vi "gui_config.vi"(0 "PS Setting":T2, 1 "LIMIT":T1, 5 "error in (no error)":errorcluster, 6 "Torque":refnum<vi>, 12 "Speed":refnum<vi>) -> (11 "Water mode":bool, 13 "Offset out":dbl, 14 "PS Setting out":T2, 15 "Set_ECU_MODE":i32, 16 "mode out":bool, 17 "LIMIT  out":T1, 18 "power mode":bool, 19 "error out":errorcluster)   [LabVIEW 2019]
uses:
  ps_setting.ctl
  LIMIT DATA.ctl
panel:
  in  "Offset":dbl
  in  "chiller":bool
  in  "ps":bool
  in  "mode":bool
  in  "Exit":bool
  in  "最高转速 [rpm]":i32
  in  "最大扭矩 [Nm]":dbl
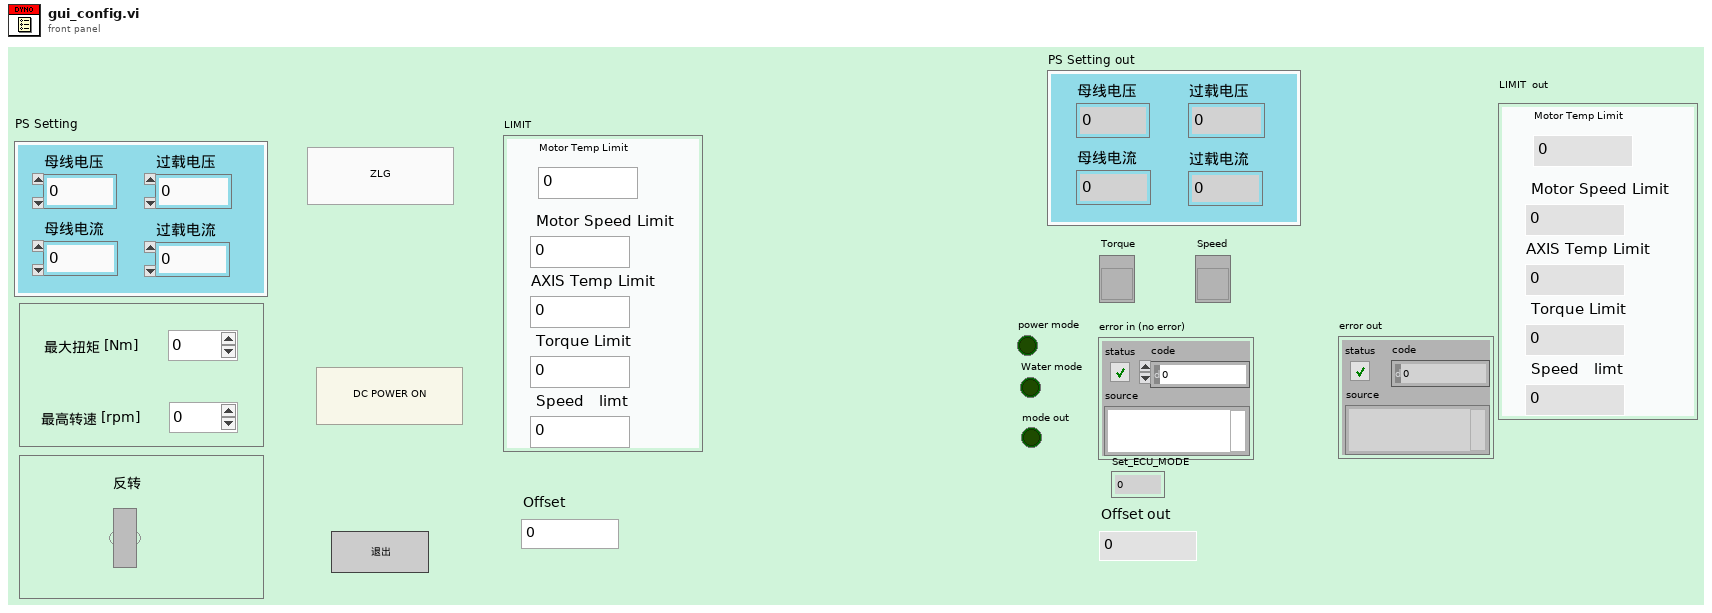
[diagram p1: front panel]
types:
  T1 = typedef "LIMIT DATA.ctl" = cluster{"Motor Temp Limit ":dbl, " Motor Speed Limit ":dbl, "AXIS Temp Limit  ":dbl, " Torque Limit":dbl, " Speed   limt":dbl}
  T2 = typedef "ps_setting.ctl" = cluster{"母线电压":sgl, "母线电流":sgl, "过载电压":sgl, "过载电流":sgl}
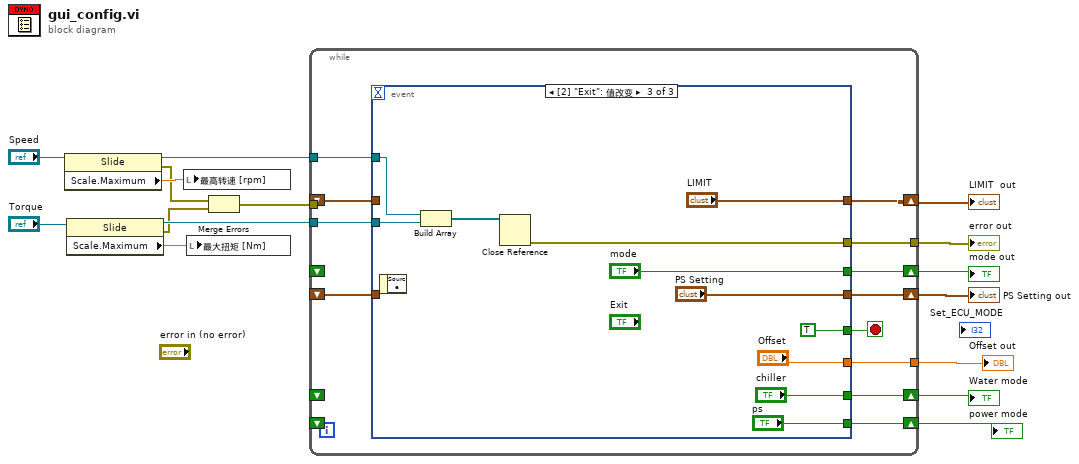
[diagram p0: block diagram]
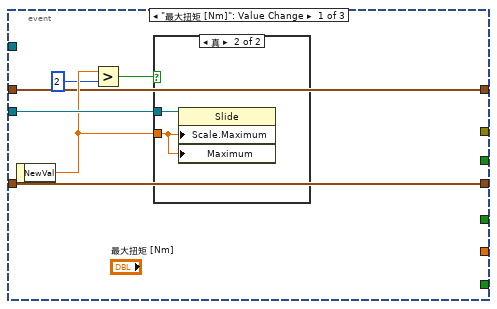
[diagram p2: hidden frame]
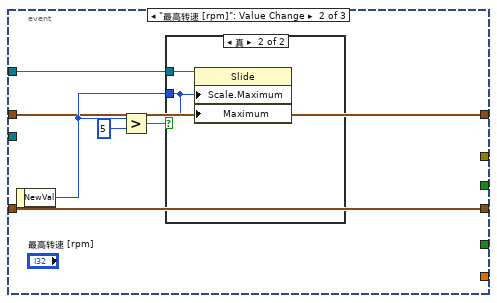
[diagram p4: hidden frame]
diagram:
  n1 = property class="Slide"(reference="Speed") -> (reference out=w12:refnum<vi>, error out=w10:errorcluster, "Scale.Maximum"=w13:dbl)  [unwired: 1 in]
  n2 = property class="Slide"(reference="Torque") -> (reference out=w15:refnum<vi>, error out=w9:errorcluster, "Scale.Maximum"=w14:dbl)  [unwired: 1 in]
  n3 = local write "最高转速 [rpm]"(w13) -> ()
  n4 = local write "最大扭矩 [Nm]"(w14) -> ()
  n5 = Merge Errors(w10, w9) -> (w6:errorcluster)
  n6 = while {
    tunnel: w15 -> [w28]
    tunnel: w12 -> [w27]
    tunnel: [w24] -> w8
    tunnel: w6 -> [_]
    shift-right: [w23] -> w5
    shift-left: _ -> [_]
    shift-right: [w22] -> w4
    shift-left: _ -> [_]
    shift-right: [w21] -> w3
    shift-left: _ -> [_]
    shift-right: [w25] -> w7
    shift-left: _ -> [w19]
    shift-right: [w20] -> w2
    shift-left: _ -> [w18]
    tunnel: [w17] -> w1
    stop <- w26 stop-if-true
    n7 = event shown="[2] \"Exit\": 值改变" {
      selector: _ -> [_ _ _]
      dyn-events: _ -> [_ _ _]
      timeout: _ -> [_ _ _]
      tunnel: w28 -> [w34 _ w54]
      tunnel: w27 -> [_ w42 w55]
      tunnel: [_ _ TRUE] -> w26
      tunnel: [_ _ w47] -> w24
      tunnel: [w29 w38 "PS Setting"] -> w25
      tunnel: [_ _ "mode"] -> w23
      tunnel: [_ _ "ps"] -> w22
      tunnel: [_ _ "chiller"] -> w21
      tunnel: [w30 w37 "LIMIT"] -> w20
      tunnel: w19 -> [w29 w38 _]
      tunnel: w18 -> [w30 w37 _]
      tunnel: [_ _ "Offset"] -> w17
      event "最大扭矩 [Nm]": Value Change {
        n8 = event-data() -> ("NewVal"=w33:dbl)  [unwired: 1 in]
        n9 = Greater?(x=w33, y=2) -> (0:w31:bool)
        n10 = case shown="真" w31 {
          tunnel: w34 -> [_ w36]
          tunnel: w33 -> [_ w35]
          frame False {
          }
          frame True {
            n11 = property class="Slide"(reference=w36, "Scale.Maximum"=w35, "Maximum"=w35) -> ()  [unwired: 1 in, 2 out]
          }
        }
      }
      event "最高转速 [rpm]": Value Change {
        n12 = event-data() -> ("NewVal"=w40:i32)  [unwired: 1 in]
        n13 = Greater?(x=w40, y=5) -> (0:w41:bool)
        n14 = case shown="真" w41 {
          tunnel: w42 -> [_ w44]
          tunnel: w40 -> [_ w43]
          frame False {
          }
          frame True {
            n15 = property class="Slide"(reference=w44, "Scale.Maximum"=w43, "Maximum"=w43) -> ()  [unwired: 1 in, 2 out]
          }
        }
      }
      event "Exit": Value Change {
        n16 = event-data() -> ()  [unwired: 1 in, 1 out]
        n17 = Build Array(w55, w54) -> (w53:refnum<vi>[])
        n18 = Close Reference(reference=w53) -> (error out=w47:errorcluster)  [unwired: 1 in]
      }
    }
  }
  "error out" <- w8
  "PS Setting out" <- w7
  "mode out" <- w5
  "power mode" <- w4
  "Water mode" <- w3
  "LIMIT  out" <- w2
  "Offset out" <- w1
